vi "General Settings GUI.vi"() -> ()   [LabVIEW 2014]
uses:
  Controls/Translation Stage Types.ctl
  Hardware/Table Stage/Controls/Translation Stage Cluster.ctl
  Controls/Queue Manager Actions.ctl
  Controls/QueueNames.ctl
  Controls/MessagePacket.ctl
panel:
  in  "Tree":string(tree)
  in  "Control Panel":T1(tab)
  in  "Table Stage Motion Controls":enum32{"Table Stage Controls"}(tab)
  in  "+Y":bool
  in  "-X":bool
  in  "+X":bool
  in  "-Y":bool
  in  "+Z":bool
  in  "-Z":bool
  in  "Mosaic Quick Nav.":bool[][](array[boolean])
  in  "X Axis":T2={"Position"=0.0, "Is.Enabled?"=FALSE, "Is.Connected?"=FALSE, "Device SN"="45876539", "AccelerationMaximum"=0.0, "VelocityMaximum"=0.0, "Acceleration"=0.0, "Velocity"=0.0, "waitTimeout (ms)"=0}
  in  "Cluster":T4
  in  "Center Galvos":bool
  in  "X Stage 4":T3 caption="Device Type"
  in  "X Stage 3":T3 caption="Device Type"
  in  "Z Axis":T2={"Position"=0.0, "Is.Enabled?"=FALSE, "Is.Connected?"=FALSE, "Device SN"="45876539", "AccelerationMaximum"=0.0, "VelocityMaximum"=0.0, "Acceleration"=0.0, "Velocity"=0.0, "waitTimeout (ms)"=0}
  in  "Y Axis":T2={"Position"=0.0, "Is.Enabled?"=FALSE, "Is.Connected?"=FALSE, "Device SN"="45876539", "AccelerationMaximum"=0.0, "VelocityMaximum"=0.0, "Acceleration"=0.0, "Velocity"=0.0, "waitTimeout (ms)"=0}
  out "Error Out":errorcluster
  in  "Error In":errorcluster
  # "Stage Controls"
  # "XYZ Axis Control"
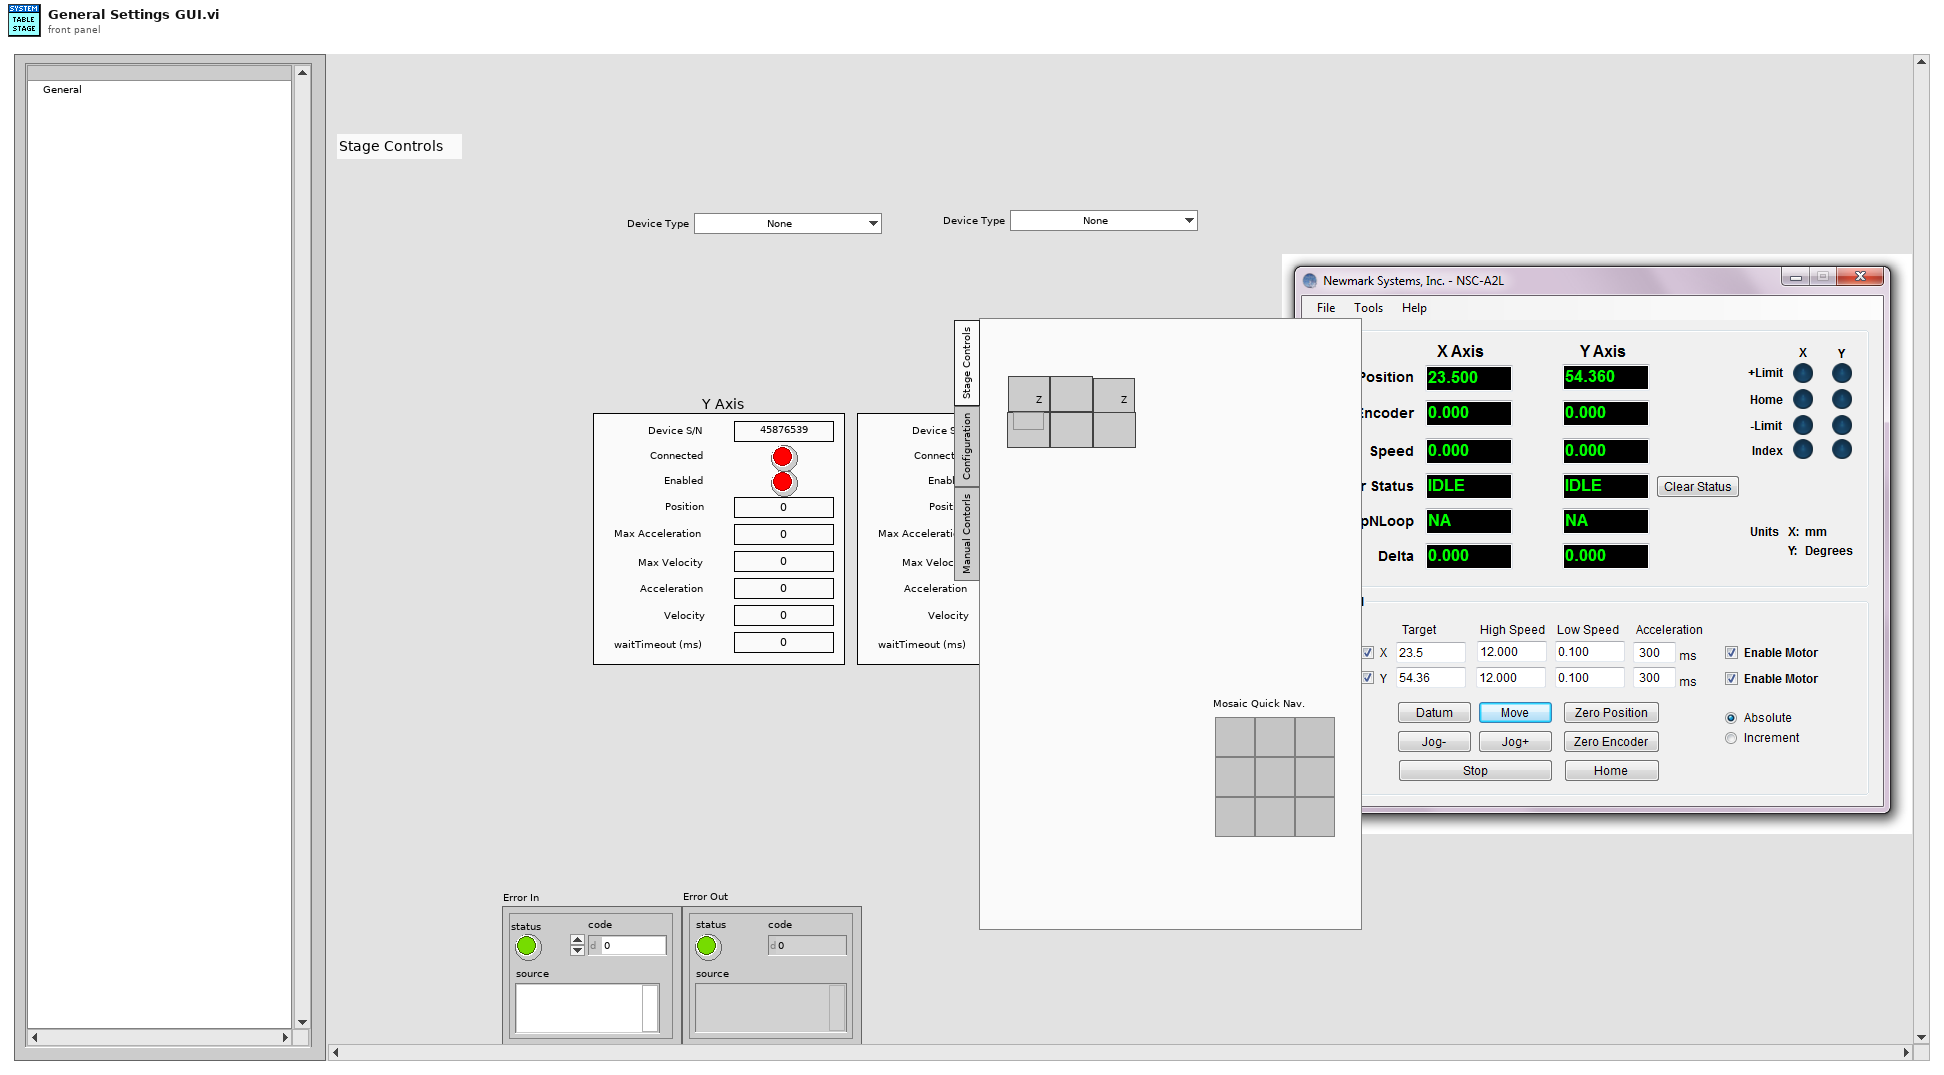
[diagram p1: front panel]
types:
  T1 = enum32{"Stage Controls", "Configuration", "Manual Contorls"}
  T2 = typedef "Translation Stage Cluster.ctl" = cluster{"Position":dbl, "Is.Enabled?":bool, "Is.Connected?":bool, "Device SN":string, "AccelerationMaximum":dbl, "VelocityMaximum":dbl, "Acceleration":dbl, "Velocity":dbl, "waitTimeout (ms)":i32}
  T3 = typedef "Translation Stage Types.ctl" = enum16{"None", "Thorlabs LTS", "Thorlabs MLJ"}
  T4 = cluster{"Home":bool, "Reconnect X":bool, "X Stage 2":T3}
  T5 = typedef "MessagePacket.ctl" = cluster{"Message":string, "Parameter":variant}
  T6 = typedef "QueueNames.ctl" = enum16{"Main GUI", "Main Scan Processor", "Main Display", "Main Table Stage GUI", "Main Table Stage Proc.", "Scan Engine"}
  T7 = typedef "Queue Manager Actions.ctl" = enum16{"Init", "Enqueue", "Enqueue All", "Preview Queue", "Dequeue", "Get Status", "Flush Queue", "Flush All Queues", "Release All Queues", "Release Queue", "Enqueue at Opposite End"}
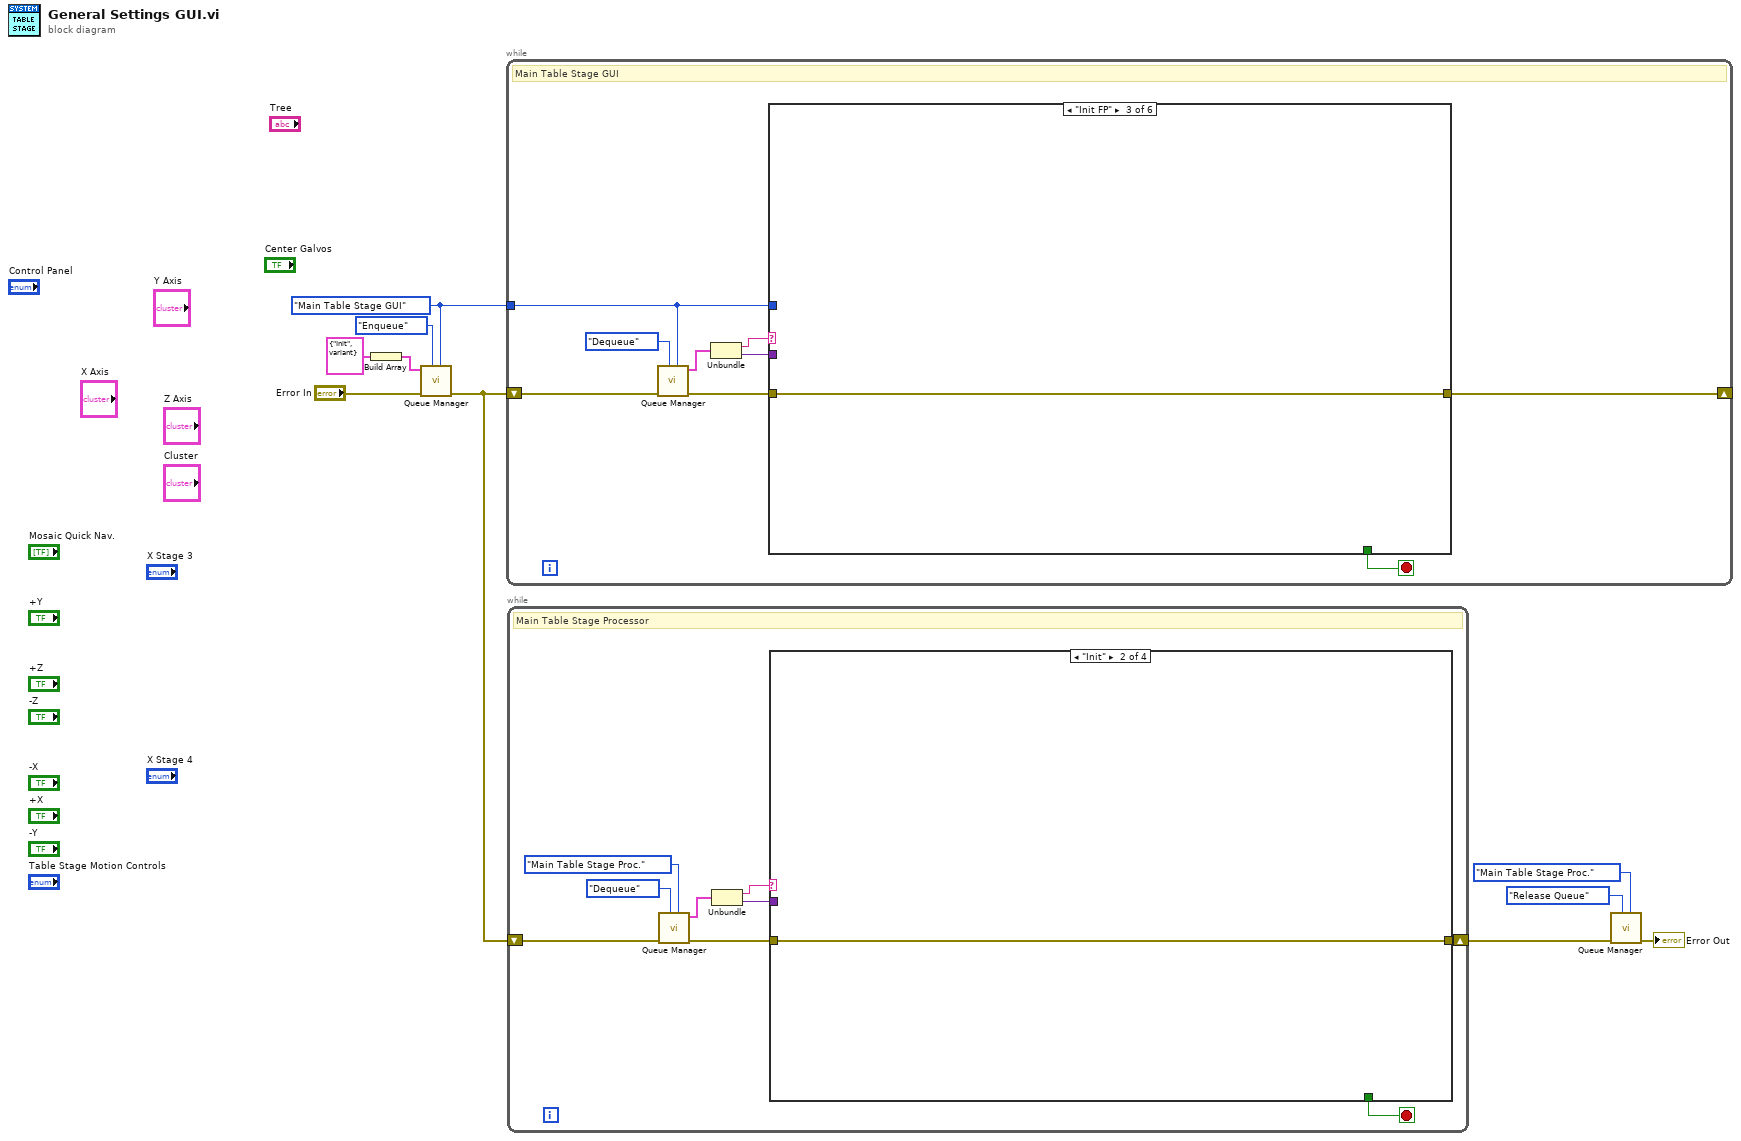
[diagram p0: block diagram]
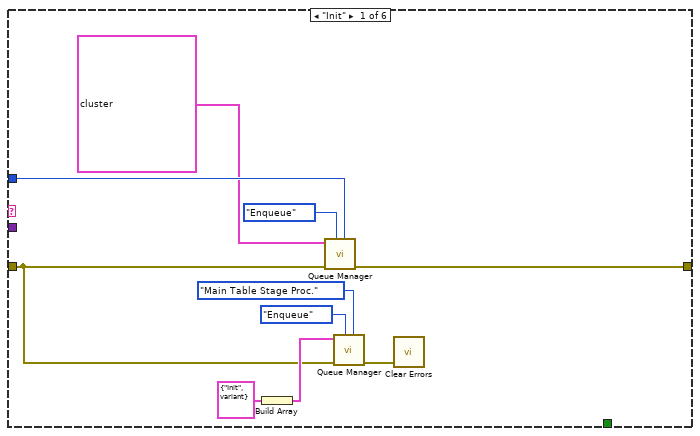
[diagram p2: hidden frame]
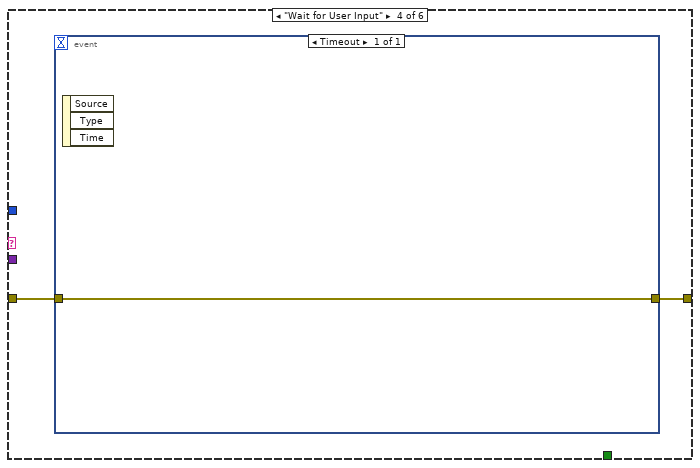
[diagram p4: hidden frame]
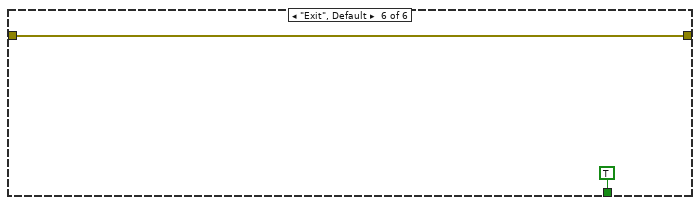
[diagram p6: hidden frame]
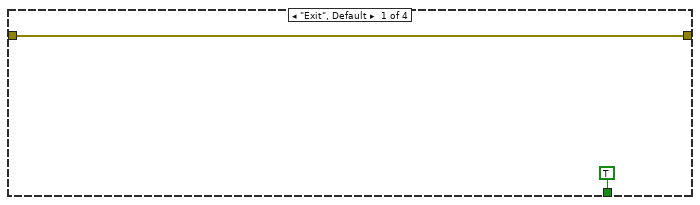
[diagram p7: hidden frame]
diagram:
  w1 = QueueNames."Main Table Stage GUI" ("Queue Name")
  n1 = Build Array(T5 {"Message"="Init", "Parameter"=variant} ("Message Packet [In]")) -> (w2:T5[])
  n2 = call "Queue Manager.vi"("Queue Name"=w1, "Action"=Queue_Manager_Actions."Enqueue", "Error In"="Error In", "Message Packet Array"=w2) -> ("Error Out"=w4:errorcluster)  [unwired: 5 in, 2 out]
  n3 = while {
    shift-right: [w12] -> _
    shift-left: w4 -> [w18]
    tunnel: w1 -> [w11]
    stop <- w13 stop-if-true
    # "Main Table Stage GUI"
    n4 = call "Queue Manager.vi"("Queue Name"=w11, "Action"=Queue_Manager_Actions."Dequeue", "Error In"=w18) -> ("Error Out"=w17:errorcluster, "Message Packet [Out]"=w16:T5)  [unwired: 6 in, 1 out]
    n5 = Unbundle(w16) -> ("Message"=w15:string, "Parameter"=w14:variant)
    n6 = case shown="\"Init FP\"" w15 {
      tunnel: w17 -> [w23 w30 w31 w33 w35 w36]
      tunnel: w14 -> [_ _ _ _ _ _]
      tunnel: [w25 w30 w31 w32 w35 w36] -> w12
      tunnel: [_ _ _ _ _ TRUE] -> w13
      tunnel: w11 -> [w22 _ _ _ _ _]
      frame "Init" {
        n7 = Build Array(T5 {"Message"="Init", "Parameter"=variant} ("Message Packet [In]")) -> (w26:T5[])
        n8 = call "Queue Manager.vi"("Queue Name"=w22, "Action"=Queue_Manager_Actions."Enqueue", "Error In"=w23, "Message Packet Array"=T5[] [{"Message"="Load Param", "Parameter"=variant}, {"Message"="Init FP", "Parameter"=variant}, {"Message"="Wait for User Input", "Parameter"=variant}]) -> ("Error Out"=w25:errorcluster)  [unwired: 5 in, 2 out]
        n9 = call "Queue Manager.vi"("Queue Name"=QueueNames."Main Table Stage Proc.", "Action"=Queue_Manager_Actions."Enqueue", "Error In"=w23, "Message Packet Array"=w26) -> ("Error Out"=w24:errorcluster)  [unwired: 5 in, 2 out]
        n10 = call <vilib>:"Clear Errors.vi"("error in (no error)"=w24) -> ()  [unwired: 5 in, 2 out]
      }
      frame "Load Param" {
      }
      frame "Init FP" {
      }
      frame "Wait for User Input" {
        n11 = event shown="[0] Timeout" {
          selector: _ -> [_]
          dyn-events: _ -> [_]
          timeout: _ -> [_]
          tunnel: w33 -> [w34]
          tunnel: [w34] -> w32
          event Timeout {
            n12 = event-data() -> ()  [unwired: 1 in, 3 out]
          }
        }
      }
      frame "Idle" {
      }
      frame "Exit", Default {
      }
    }
  }
  n13 = while {
    shift-right: [w39] -> w10
    shift-left: w4 -> [w44]
    stop <- w38 stop-if-true
    # "Main Table Stage Processor"
    n14 = call "Queue Manager.vi"("Queue Name"=QueueNames."Main Table Stage Proc.", "Action"=Queue_Manager_Actions."Dequeue", "Error In"=w44) -> ("Error Out"=w43:errorcluster, "Message Packet [Out]"=w42:T5)  [unwired: 6 in, 1 out]
    n15 = Unbundle(w42) -> ("Message"=w41:string, "Parameter"=w40:variant)
    n16 = case shown="\"Init\"" w41 {
      tunnel: w43 -> [w47 w49 w50 w51]
      tunnel: w40 -> [_ _ _ _]
      tunnel: [w47 w49 w50 w51] -> w39
      tunnel: [TRUE _ _ _] -> w38
      frame "Exit", Default {
      }
      frame "Init" {
      }
      frame "Init Hardware" {
      }
      frame "Idle" {
      }
    }
  }
  n17 = call "Queue Manager.vi"("Queue Name"=QueueNames."Main Table Stage Proc.", "Action"=Queue_Manager_Actions."Release Queue", "Error In"=w10) -> ("Error Out"=→"Error Out":errorcluster)  [unwired: 6 in, 2 out]
